vi "ConfigurateDatabase.vi"() -> (5 "Logging interval":dbl)   [LabVIEW 2021]
panel:
  in  "stop":bool
  out "subarray":string[](array[string])
  out "Data 2":string[][](array[string])
  out "error out":errorcluster
  in  "error in (no error)":errorcluster
  in  "Update interval":bool
  in  "Update unit":bool
  in  "tag_id":dbl
  in  "Measurement interval":dbl
  in  "Measurement interval unit":string
  in  "Measurement unit":string
  # "Station_id"
  # "Unit"
  # "Name"
  # "Description"
  # "Interval"
  # "Unit"
  # "Tag_id"
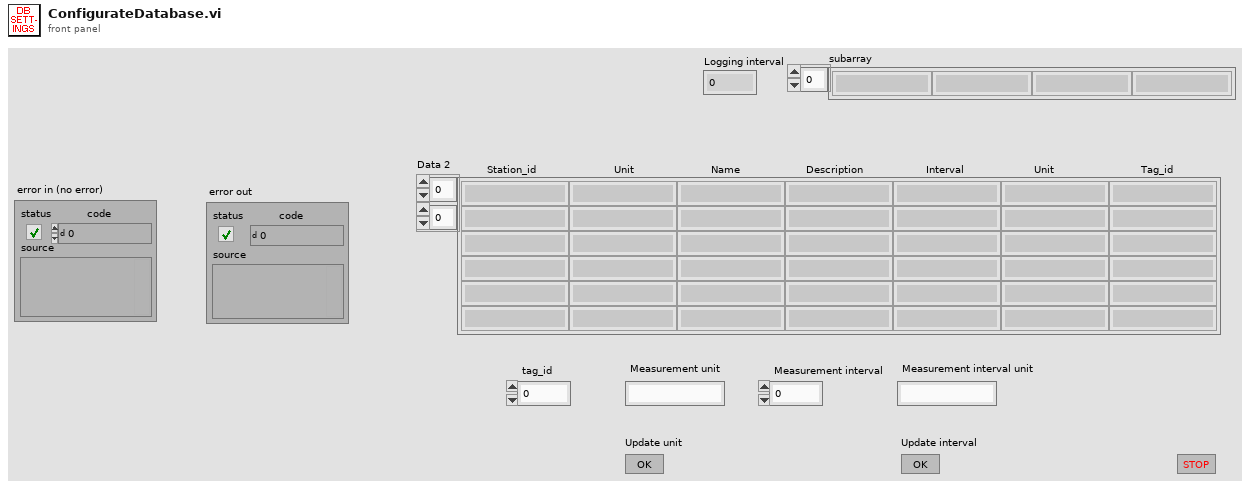
[diagram p1: front panel]
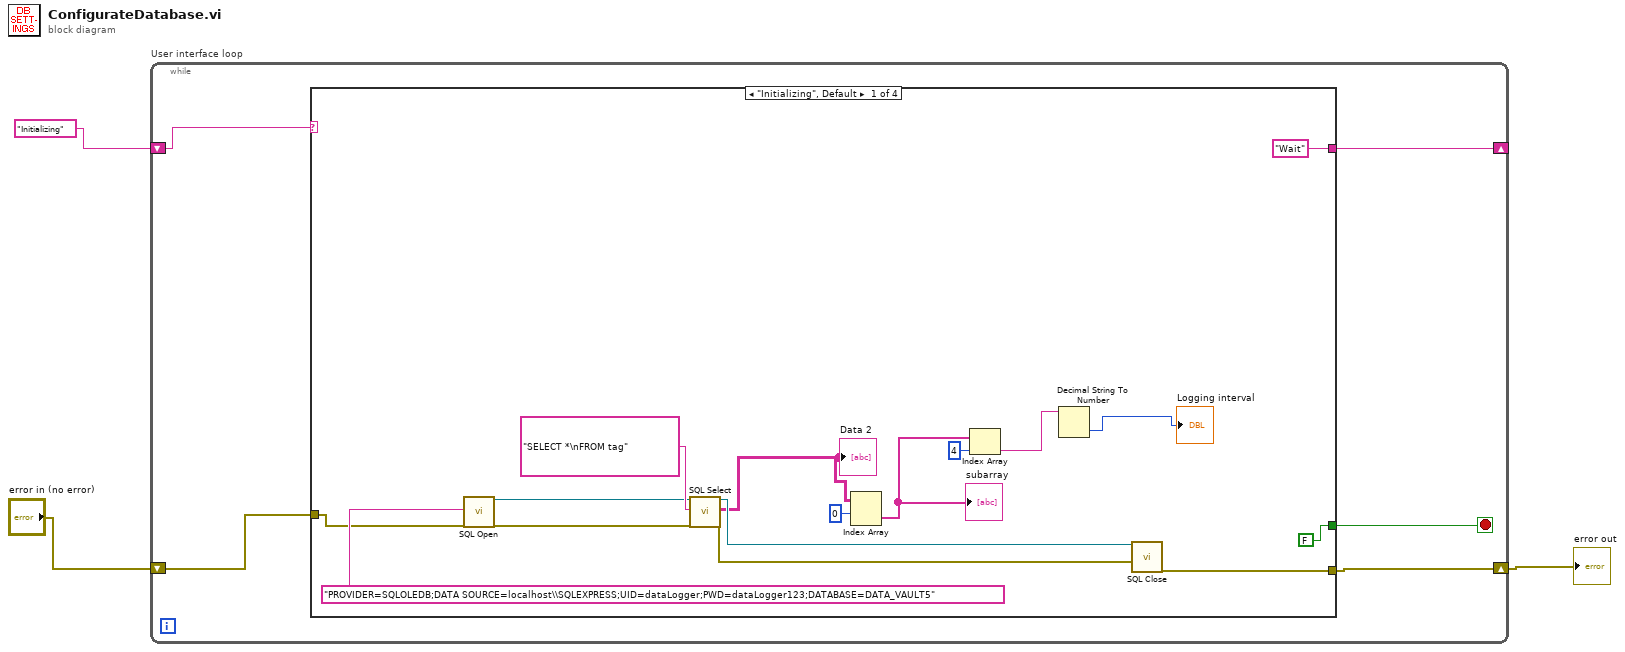
[diagram p0: block diagram]
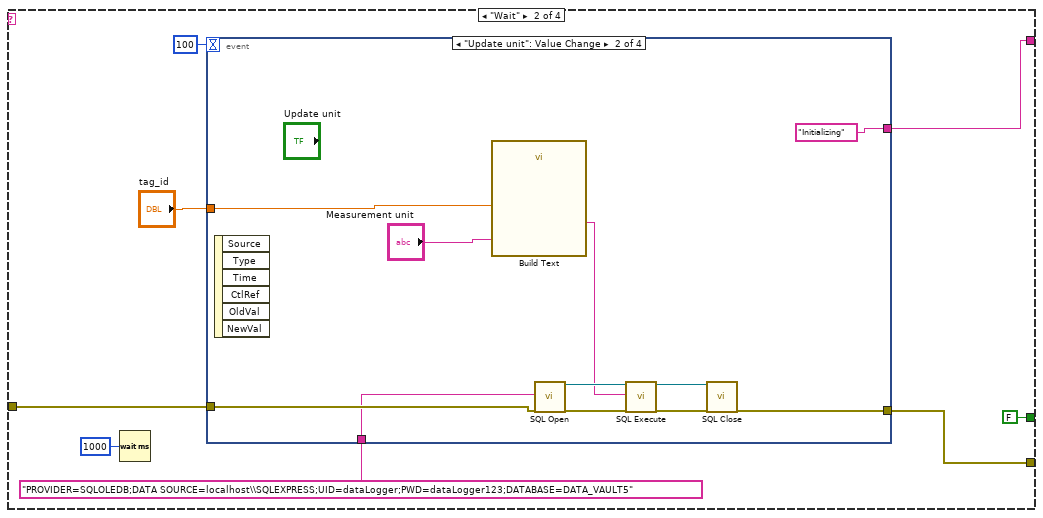
[diagram p2: hidden frame]
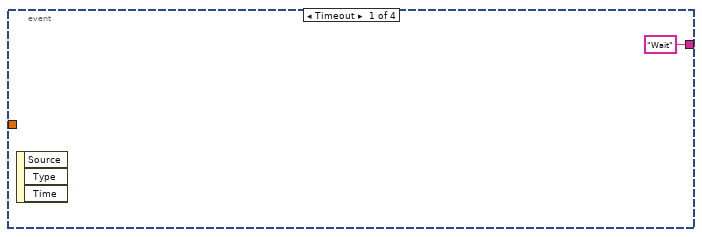
[diagram p3: hidden frame]
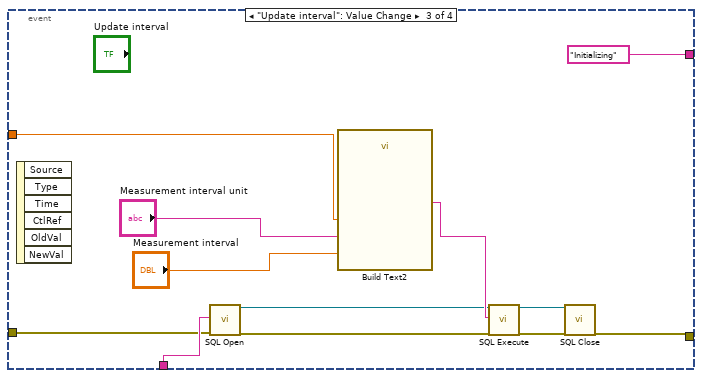
[diagram p4: hidden frame]
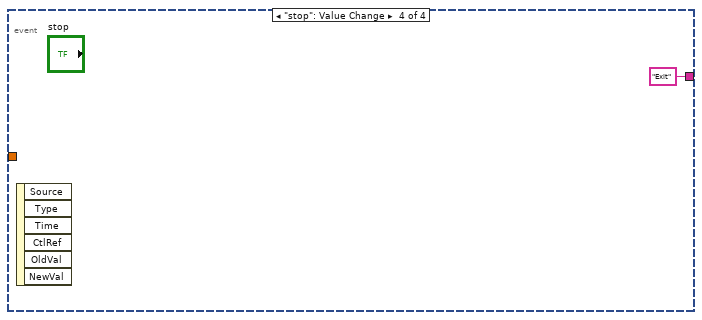
[diagram p5: hidden frame]
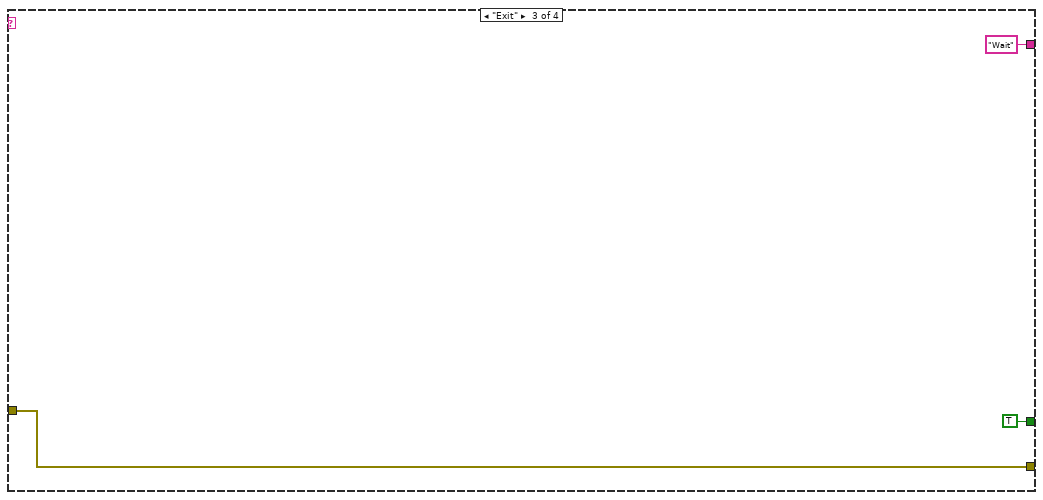
[diagram p6: hidden frame]
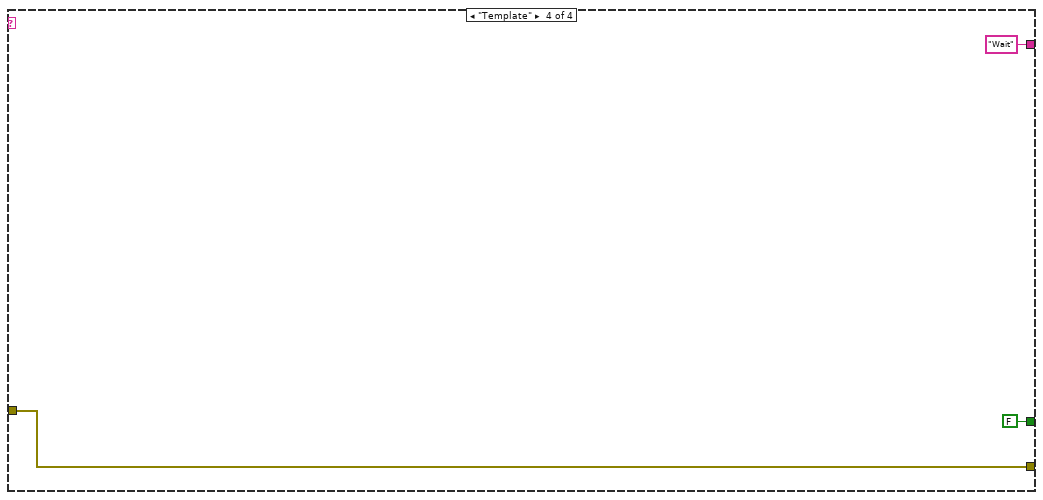
[diagram p7: hidden frame]
diagram:
  n1 = while "User interface loop" {
    shift-right: [w7] -> _
    shift-left: "Initializing" -> [w8]
    shift-right: [w4] -> w1
    shift-left: "error in (no error)" -> [w5]
    stop <- w6 stop-if-true
    n2 = case shown="\"Initializing\", Default" w8 {
      tunnel: ["Wait" w27 "Wait" "Wait"] -> w7
      tunnel: [FALSE FALSE TRUE FALSE] -> w6
      tunnel: w5 -> [w21 w31 w58 w61]
      tunnel: [w18 w30 w58 w61] -> w4
      frame "Initializing", Default {
        n3 = call <vilib>:"SQL Open.vi"("ConnectionString In"="PROVIDER=SQLOLEDB;DATA SOURCE=localhost\\SQLEXPRESS;UID=dataLogger;PWD=dataLogger123;DATABASE=DATA_VAULT5", "Error in (no error)"=w21) -> ("Connection Out"=w16:refnum<k7>, "Error out"=w20:errorcluster)  [unwired: 16 in]
        n4 = call <vilib>:"SQL Select.vi"("Connection In"=w16, "SQL Query"="SELECT *\nFROM tag", "Error in (no error)"=w20) -> ("Connection Out"=w15:refnum<k7>, "Data"=w14:string[][], "Error out"=w19:errorcluster)  [unwired: 14 in]
        "Data 2" <- w14
        n5 = Index Array(array=w14, index (row)=0) -> (element=w12:string[])  [unwired: 1 in]
        "subarray" <- w12
        n6 = Index Array(array=w12, index=4) -> (element=w10:string)
        n7 = Decimal String To Number(string=w10) -> (number=→"Logging interval":i32)  [unwired: 2 in, 1 out]
        n8 = call <vilib>:"SQL Close.vi"("Connection In"=w15, "Error in (no error)"=w19) -> ("Error out"=w18:errorcluster)  [unwired: 17 in]
      }
      frame "Wait" {
        n9 = Wait (ms)(milliseconds to wait=u32 1000) -> ()  [unwired: 1 out]
        n10 = event shown="[1] \"Update unit\": Value Change" {
          selector: _ -> [_ _ _ _]
          dyn-events: _ -> [_ _ _ _]
          timeout: 100 -> [_ _ _ _]
          tunnel: w31 -> [_ w38 w47 _]
          tunnel: [_ w37 w46 _] -> w30
          tunnel: "PROVIDER=SQLOLEDB;DATA SOURCE=localhost\\SQLEXPRESS;UID=dataLogger;PWD=dataLogger123;DATABASE=DATA_VAULT5" ("ConnectionString In") -> [_ w36 w48 _]
          tunnel: "tag_id" -> [_ w35 w49 _]
          tunnel: ["Wait" "Initializing" "Initializing" "Exit"] -> w27
          event Timeout {
            n11 = event-data() -> ()  [unwired: 1 in, 3 out]
          }
          event "Update unit": Value Change {
            n12 = event-data() -> ()  [unwired: 1 in, 6 out]
            n13 = call "Build Text"("tag_id"=w35, "measurement_unit"="Measurement unit") -> ("Result"=w42:string)  [unwired: 12 in, 1 out]
            n14 = call <vilib>:"SQL Open.vi"("ConnectionString In"=w36, "Error in (no error)"=w38) -> ("Connection Out"=w44:refnum<k7>, "Error out"=w43:errorcluster)  [unwired: 16 in]
            n15 = call <vilib>:"SQL Execute.vi"("Connection In"=w44, "SQL Query"=w42, "Error in (no error)"=w43) -> ("Connection Out"=w40:refnum<k7>, "Error out"=w41:errorcluster)  [unwired: 15 in]
            n16 = call <vilib>:"SQL Close.vi"("Connection In"=w40, "Error in (no error)"=w41) -> ("Error out"=w37:errorcluster)  [unwired: 17 in]
          }
          event "Update interval": Value Change {
            n17 = event-data() -> ()  [unwired: 1 in, 6 out]
            n18 = call <vilib>:"SQL Open.vi"("ConnectionString In"=w48, "Error in (no error)"=w47) -> ("Connection Out"=w52:refnum<k7>, "Error out"=w53:errorcluster)  [unwired: 16 in]
            n19 = call "Build Text2"("tag_id"=w49, "measurement_interval_unit"="Measurement interval unit", "measurement_interval"="Measurement interval") -> ("Result"=w56:string)  [unwired: 11 in, 1 out]
            n20 = call <vilib>:"SQL Execute.vi"("Connection In"=w52, "SQL Query"=w56, "Error in (no error)"=w53) -> ("Connection Out"=w54:refnum<k7>, "Error out"=w55:errorcluster)  [unwired: 15 in]
            n21 = call <vilib>:"SQL Close.vi"("Connection In"=w54, "Error in (no error)"=w55) -> ("Error out"=w46:errorcluster)  [unwired: 17 in]
          }
          event "stop": Value Change {
            n22 = event-data() -> ()  [unwired: 1 in, 6 out]
          }
        }
      }
      frame "Exit" {
      }
      frame "Template" {
      }
    }
  }
  "error out" <- w1
